vi "addModulePath.vi"(8 "error in (no error)":errorcluster, 10 "modulePathStr":string, 11 "IInstanceBuilder in":refnum<class "IInstanceBuilder.lvclass">) -> (0 "error out":errorcluster, 3 "IInstanceBuilder out":refnum<class "IInstanceBuilder.lvclass">)   [LabVIEW 2022 SP3, in "openDAQ.lvlib" / "IBaseObject.lvlib" / "IInstanceBuilder.lvlib" / "IInstanceBuilder.lvclass"]
uses:
  <instrlib>/openDAQ/Public/Classes/IInstanceBuilder/IInstanceBuilder.lvclass
  <instrlib>/openDAQ/Public/Classes/IInstanceBuilder/IInstanceBuilder.lvclass/IInstanceBuilder.ctl
  <instrlib>/openDAQ/Public/Classes/daqCoreTypes/IString/IString.lvclass
  <instrlib>/openDAQ/Binaries/Windows/x86/copendaq32.dll
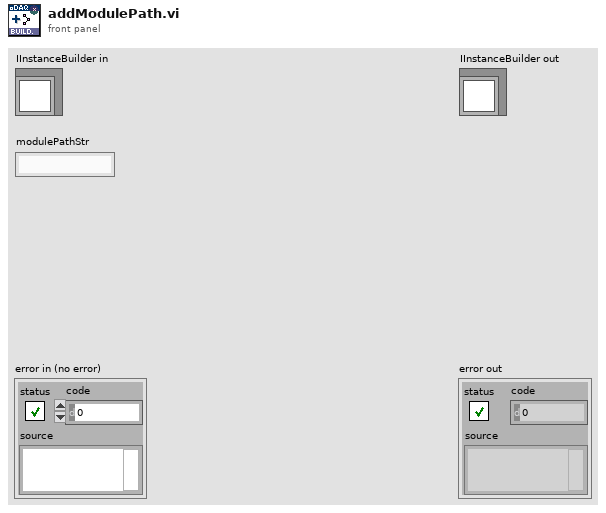
[diagram p1: front panel]
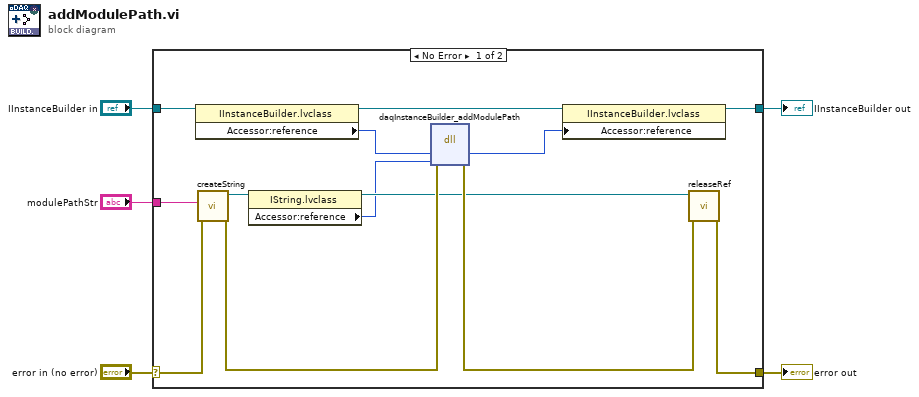
[diagram p0: block diagram]
diagram:
  n1 = case shown="No Error" "error in (no error)" {
    selector: "error in (no error)" -> [w17 w20]
    tunnel: [w6 w20] -> w4
    tunnel: [w10 w19] -> w2
    tunnel: "IInstanceBuilder in" -> [w11 w19]
    tunnel: "modulePathStr" -> [w18 _]
    frame No Error {
      n2 = property class="IInstanceBuilder.lvclass"(reference=w11) -> (reference out=w9:refnum<class "IInstanceBuilder.lvclass">, "Accessor:reference"=w8:i64)  [unwired: 1 in, 1 out]
      n3 = call <instrlib>:"createString.vi"("error in (no error)"=w17, "String"=w18) -> ("error out"=w15:errorcluster, "IString out"=w14:refnum<class "IString.lvclass">)  [unwired: 8 in]
      n4 = property class="IString.lvclass"(reference=w14) -> (reference out=w13:refnum<class "IString.lvclass">, "Accessor:reference"=w12:i64)  [unwired: 1 in, 1 out]
      n5 = dll-call lib="C:/Program Files (x86)/National Instruments/LabVIEW 2022/instr.lib/openDAQ/Binaries/Windows/x86/copendaq*.*" fn="daqInstanceBuilder_addModulePath"(error in=w15, "instanceBuilder"=w8, "modulePath"=w12) -> (error out=w16:errorcluster, "instanceBuilder"=w7:i64)  [unwired: 4 in, 1 out]
      n6 = property class="IInstanceBuilder.lvclass"(reference=w9, "Accessor:reference"=w7) -> (reference out=w10:refnum<class "IInstanceBuilder.lvclass">)  [unwired: 1 in, 1 out]
      n7 = call-dynamic "releaseRef.vi"("error in (no error)"=w16, "IBaseObject in"=w13) -> ("error out"=w6:errorcluster)  [unwired: 9 in]
    }
    frame Error {
    }
  }
  "error out" <- w4
  "IInstanceBuilder out" <- w2
